vi "lab3b_part2_signal2.vi"() -> ()   [LabVIEW 2019]
uses:
  <vilib>/Platform/TimedLoop/XDataNode/timing_clust.ctl
  <vilib>/Platform/TimedLoop/XDataNode/nitl_modes.ctl
  <vilib>/Platform/TimedLoop/XDataNode/wakeup.ctl
  <vilib>/Analysis/3filter.llb/Filter Passband Type.ctl
  <vilib>/DAQmx/write.llb/DAQmx Write (Analog DBL 1Chan 1Samp).vi
  <vilib>/DAQmx/read.llb/DAQmx Read (Analog DBL 1Chan 1Samp).vi
  <vilib>/DAQmx/create/channels.llb/DAQmx Create Channel (AO-Voltage-Basic).vi
  <vilib>/DAQmx/miscellaneous.llb/DAQmx Fill In Error Info.vi
  <vilib>/DAQmx/create/channels.llb/DAQmx Create Channel (AI-Voltage-Basic).vi
  <vilib>/platform/TimedLoop/XDataNode/XDataNode.xnode
  <vilib>/Platform/TimedLoop/XDataNode/XDNodeRunTimeDep.lvlib
  <vilib>/Analysis/NI_AALBase.lvlib
  <vilib>/ptbypt/NI_PtbyPt.lvlib
panel:
  in  "Position low cutoff freq: fl":dbl=0.125 format="%0.3f"
  out "Waveform Chart":cluster{"data":dbl, dbl}(graph)
  in  "PID On/Off":bool
  in  "PID gains":cluster{"Kp":dbl, "Ki":dbl, "Kd":dbl}
  out "Voltage 2":dbl(graph)
  out "Voltage":dbl
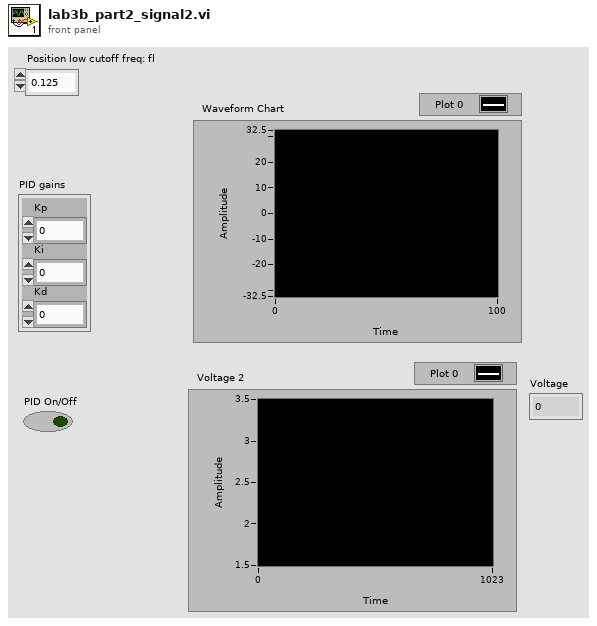
[diagram p1: front panel]
types:
  T1 = typedef "NI_AALBase.lvlib/Filter Passband Type.ctl" = enum32{"Lowpass", "Highpass", "Bandpass", "Bandstop"}
  T2 = typedef "XDNodeRunTimeDep.lvlib/timing_clust.ctl" = cluster{"Expected End [f-1]":u64, "Actual End [f-1]":u64, "Finished Late? [f-1]":bool, "Expected End [i-1]":u64, "Actual End [i-1]":u64, "Finished Late? [i-1]":bool, "Expected Start [i]":u64, "Actual Start [i]":u64, "Expected Start [f]":u64, "Actual Start [f]":u64, "Source Name":string, "Structure Name":string, "Period":i64, "Deadline":i64, "Offset":i64, "Start":i64, "Priority":i32, "Timeout":i32, "Mode":T3, "Wakeup Reason":T4, "Error":errorcluster, "Source Type":string, "Secondary Source Type":string, "Global End Time":u64, "Global Start Time":u64, "Frame Duration":u64, "Iteration Duration":u64, "Assigned CPU":i32, "I/O Scan Engine Mode":u32}
  T3 = typedef "XDNodeRunTimeDep.lvlib/nitl_modes.ctl" = enum32{"No Change", "Process missed periods, maintain original phase", "Discard missed periods, maintain original phase", "Process missed periods, ignore original phase", "Discard missed periods, ignore original phase"}
  T4 = typedef "XDNodeRunTimeDep.lvlib/wakeup.ctl" = enum32{"Normal", "Aborted", "Asynchronous wakeup", "Timing source error", "Timed loop error", "Timeout"}
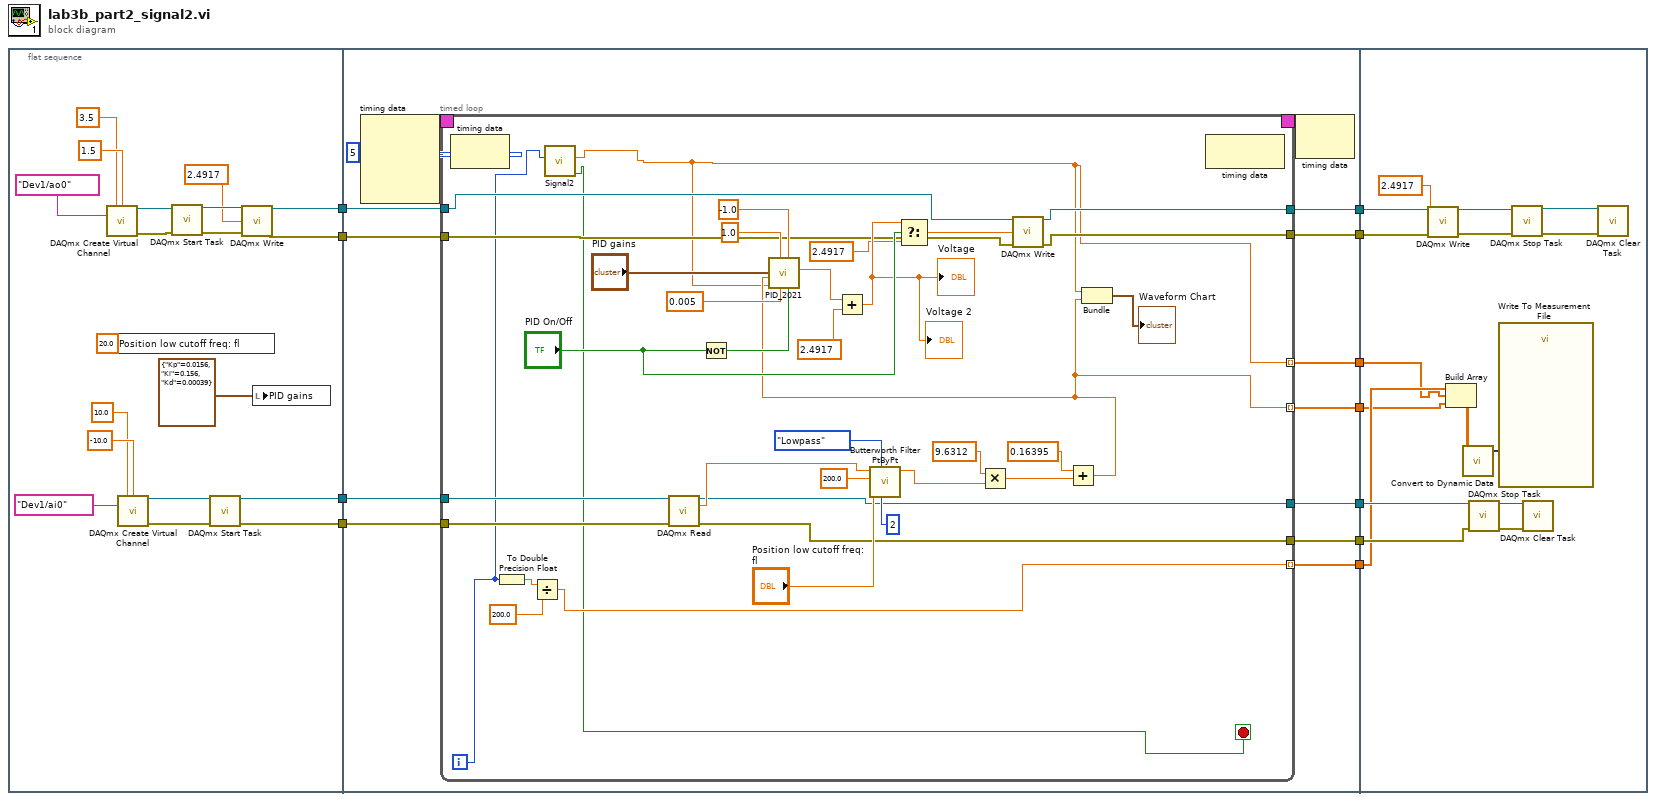
[diagram p0: block diagram]
diagram:
  n1 = flat-sequence {
    tunnel: [w22] -> w11
    tunnel: [w21] -> w10
    tunnel: [w16] -> w9
    tunnel: [w15] -> w8
    tunnel: w11 -> [w41]
    tunnel: w10 -> [w40]
    tunnel: w9 -> [w39]
    tunnel: w8 -> [w38]
    tunnel: [w37] -> w7
    tunnel: [w36] -> w6
    tunnel: [w35] -> w5
    tunnel: [w34] -> w4
    tunnel: [w33] -> w3
    tunnel: [w32] -> w2
    tunnel: [w31] -> w1
    tunnel: w7 -> [w95]
    tunnel: w6 -> [w94]
    tunnel: w5 -> [w93]
    tunnel: w4 -> [w92]
    tunnel: w3 -> [w90]
    tunnel: w2 -> [w89]
    tunnel: w1 -> [w91]
    frame #0 {
      n2 = local write "Position low cutoff freq: fl"(20.0 ("low cutoff freq: fl")) -> ()
      n3 = call-poly <vilib>:"DAQmx Create Virtual Channel.vi"("maximum value"=3.5, "minimum value"=1.5, "physical channels"=tag "Dev1/ao0") -> ("task out"=w30:refnum<k21>, "error out"=w28:errorcluster)  [unwired: 11 in]
      n4 = call-poly <vilib>:"DAQmx Create Virtual Channel.vi"("maximum value"=10.0, "minimum value"=-10.0, "physical channels"=tag "Dev1/ai0") -> ("task out"=w20:refnum<k21>, "error out"=w19:errorcluster)  [unwired: 11 in]
      n5 = call <vilib>:"DAQmx Start Task.vi"("task/channels in"=w30, "error in"=w28) -> ("task out"=w29:refnum<k21>, "error out"=w27:errorcluster)  [unwired: 12 in]
      n6 = call <vilib>:"DAQmx Start Task.vi"("task/channels in"=w20, "error in"=w19) -> ("task out"=w16:refnum<k21>, "error out"=w15:errorcluster)  [unwired: 12 in]
      n7 = call-poly <vilib>:"DAQmx Write.vi"("task/channels in"=w29, "data"=2.4917, "error in"=w27) -> ("task out"=w22:refnum<k21>, "error out"=w21:errorcluster)  [unwired: 10 in, 1 out]
      n8 = local write "PID gains"(cluster{"Kp":dbl, "Ki":dbl, "Kd":dbl} {"Kp"=0.0156, "Ki"=0.156, "Kd"=0.00039} ("PID gains")) -> ()
    }
    frame #1 {
      n9 = node-c288(i64 5 ("Period")) -> (w44:T2)  [unwired: 3 in]
      n10 = timed-loop {
        timing: w44 -> [_]
        timing-out: [_] -> w43
        tunnel: w41 -> [w55]
        tunnel: w40 -> [w54]
        tunnel: w39 -> [w80]
        tunnel: w38 -> [w79]
        tunnel: [w69] -> w37
        tunnel: [w68] -> w36
        tunnel: [w53] -> w35
        tunnel: [w52] -> w34
        tunnel: [w47] -> w33 mode=indexing
        tunnel: [w51] -> w32 mode=indexing
        tunnel: [w48] -> w31 mode=indexing
        i -> [w46]
        stop <- w45 stop-if-true
        n11 = node-c288() -> ()  [unwired: 1 in, 1 out]
        n12 = To Double Precision Float(number=w46) -> (double precision float=w50:dbl)
        n13 = Divide(x=w50, y=200.0) -> (x/y=w48:dbl)
        n14 = call "Signal2.vi"("Iteration"=w46) -> ("Stop Loop"=w45:bool, "Output"=w47:dbl)  [unwired: 9 in]
        n15 = call-poly <vilib>:"DAQmx Read.vi"("task/channels in"=w80, "error in"=w79) -> ("task out"=w69:refnum<k21>, "data"=w72:dbl, "error out"=w68:errorcluster)  [unwired: 11 in]
        n16 = Not(x="PID On/Off") -> (.not. x?=w60:bool)
        n17 = call <vilib>:"Butterworth Filter PtByPt.vi"("order"=2, "filter type"=Filter_Passband_Type."Lowpass", "low cutoff freq: fl"="Position low cutoff freq: fl", "sampling freq: fs"=200.0, "x"=w72) -> ("Filtered x"=w73:dbl)  [unwired: 4 in, 1 out]
        n18 = Multiply(x=9.6312, y=w73) -> (x*y=w75:dbl)
        n19 = Add(x=0.16395, y=w75) -> (x+y=w51:dbl)
        n20 = call "PID_2021.vi"("Reset"=w60, "Lower limit"=-1.0, "dt (s)"=0.005, "Upper limit"=1.0, "Setpoint"=w47, "Process Variable"=w51, "PID gains"="PID gains") -> ("u(t)"=w62:dbl)  [unwired: 4 in]
        n21 = Add(x=w62, y=2.4917) -> (x+y=w58:dbl)
        "Voltage 2" <- w58
        "Voltage" <- w58
        n22 = Select(t=w58, s="PID On/Off", f=2.4917) -> (s? t:f=w57:dbl)
        n23 = call-poly <vilib>:"DAQmx Write.vi"("task/channels in"=w55, "data"=w57, "error in"=w54) -> ("task out"=w53:refnum<k21>, "error out"=w52:errorcluster)  [unwired: 10 in, 1 out]
        n24 = Bundle("Output"=w47, w51) -> (→"Waveform Chart":cluster{"Output":dbl, dbl})  [unwired: 1 in]
        n25 = node-c288() -> ()  [unwired: 1 in, 1 out]
      }
      n26 = node-c288(w43) -> ()  [unwired: 1 out]
    }
    frame #2 {
      n27 = call-poly <vilib>:"DAQmx Write.vi"("task/channels in"=w93, "data"=2.4917, "error in"=w92) -> ("task out"=w102:refnum<k21>, "error out"=w99:errorcluster)  [unwired: 10 in, 1 out]
      n28 = Build Array(w91, w90, w89) -> (w88:dbl[][])
      n29 = call "Convert to Dynamic Data"("2D Array"=w88) -> ("Dynamic Data Type"=w87:dynamicdata)  [unwired: 3 in]
      n30 = call <vilib>:"DAQmx Stop Task.vi"("task/channels in"=w95, "error in"=w94) -> ("task out"=w97:refnum<k21>, "error out"=w96:errorcluster)  [unwired: 12 in]
      n31 = call "Write To Measurement File"("Signals"=w87) -> ()  [unwired: 16 in, 3 out]
      n32 = call <vilib>:"DAQmx Stop Task.vi"("task/channels in"=w102, "error in"=w99) -> ("task out"=w101:refnum<k21>, "error out"=w100:errorcluster)  [unwired: 12 in]
      n33 = call <vilib>:"DAQmx Clear Task.vi"("task in"=w97, "error in"=w96) -> ()  [unwired: 13 in, 1 out]
      n34 = call <vilib>:"DAQmx Clear Task.vi"("task in"=w101, "error in"=w100) -> ()  [unwired: 13 in, 1 out]
    }
  }
